vi "VGap_Gap Increase.vi"() -> ()   [LabVIEW 2010]
panel:
  out "error out":errorcluster
  in  "Step Increase (um)":i32
  in  "Gap Increase (um)":i32
  in  "error in (no error)":errorcluster
  in  "MCS System Locator":string
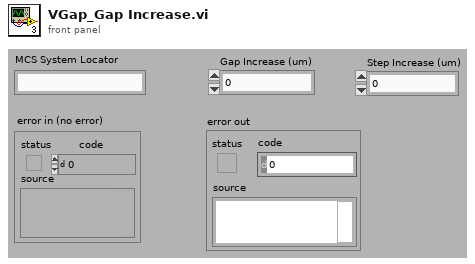
[diagram p1: front panel]
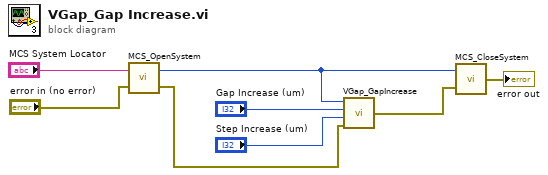
[diagram p0: block diagram]
diagram:
  n1 = call "MCS_OpenSystem.vi"("error in (no error)"="error in (no error)", "MCS System Locator"="MCS System Locator") -> ("error out"=w6:errorcluster, "System Index Out"=w5:u32)
  n2 = call "VGap_GapIncrease.vi"("error in (no error)"=w6, "Step Increase (um)"="Step Increase (um)", "Gap Increase (um)"="Gap Increase (um)", "System Index In"=w5) -> ("error out"=w4:errorcluster)
  n3 = call "MCS_CloseSystem.vi"("error in (no error)"=w4, "System Index In"=w5) -> ("error out"=→"error out":errorcluster)
